vi "API Demo.vi"() -> ()   [LabVIEW 2020]
doc: "Demonstration of API useage."
uses:
  Framework/Execution API/Execution API.lvclass
panel:
  out "All Passed?":bool
  out "Output":string
  in  "Run Tests In Parallel? (T)":bool=TRUE
  in  "Tab Control":enum32{"Path", "App Instance"}(tab)
  in  "Project, Library, or Test Class Path":path
  out "error out":errorcluster
  in  "error in":errorcluster
  # "1. Select which method you want to use for finding tests to run from the API by choosing a tab in the tab control.\n2. Fill in the path to the test to run.  \n3. Run this VI."
  # "Execute all tests found in the current application instance"
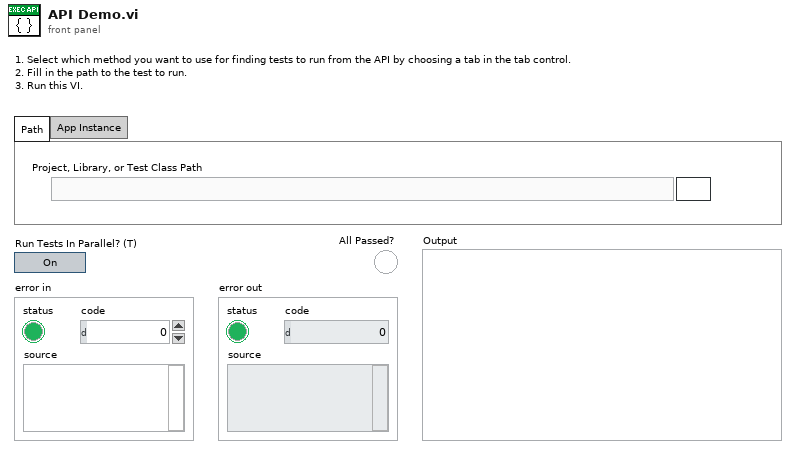
[diagram p1: front panel]
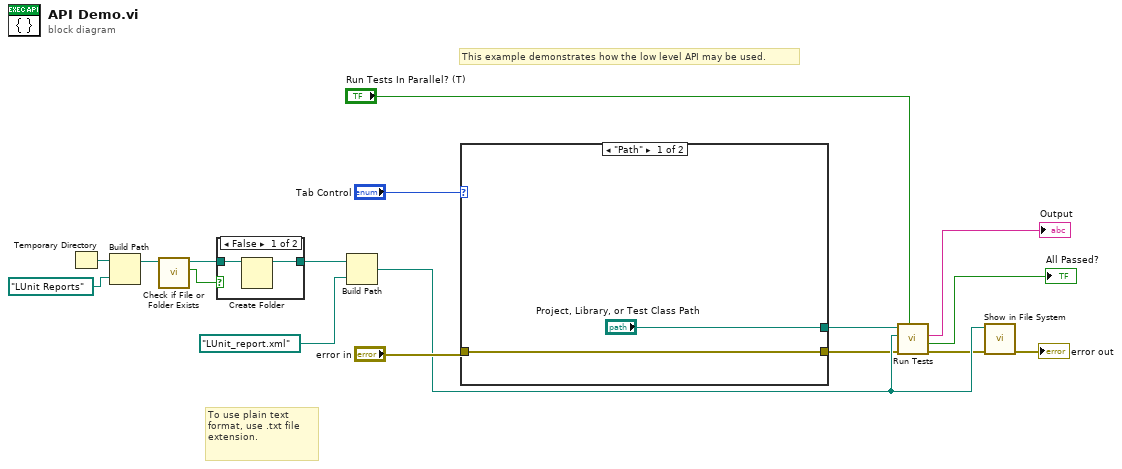
[diagram p0: block diagram]
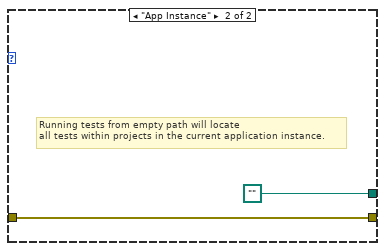
[diagram p2: hidden frame]
diagram:
  # "To use plain text format, use .txt file extension."
  # "This example demonstrates how the low level API may be used."
  n1 = Temporary Directory() -> (w12:path)
  n2 = Build Path(base path=w12, name or relative path=path "LUnit Reports") -> (appended path=w13:path)
  n3 = call <vilib>:"Check if File or Folder Exists.vi"("path"=w13) -> ("file or folder exists?"=w9:bool, "dup path"=w10:path)  [unwired: 8 in, 1 out]
  n4 = case shown="False" w9 {
    tunnel: w10 -> [w19 w20]
    tunnel: [w18 w20] -> w8
    frame False {
      n5 = Create Folder(path (use dialog)=w19) -> (created path=w18:path)  [unwired: 2 in, 2 out]
    }
    frame True {
    }
  }
  n6 = Build Path(base path=w8, name or relative path=path "LUnit_report.xml") -> (appended path=w6:path)
  n7 = case shown="\"Path\"" "Tab Control" {
    tunnel: "error in" -> [w22 w24]
    tunnel: [w22 w24] -> w3
    tunnel: ["Project, Library, or Test Class Path" path "" ("Project or Class Path")] -> w7
    frame "Path" {
    }
    frame "App Instance" {
      # "Running tests from empty path will locate\nall tests within projects in the current application instance."
    }
  }
  n8 = call "Run Tests.vi"("Run Tests In Parallel? (T)"="Run Tests In Parallel? (T)", "error in (no error)"=w3, "Report Output path"=w6, "Project, Library, or Test Class Path"=w7) -> ("error out"=w4:errorcluster, "All Passed?"=→"All Passed?":bool, "Output"=→"Output":string)  [unwired: 5 in]
  n9 = call <vilib>:"Show in File System.vi"("error in (no error)"=w4, "file or directory path"=w6) -> ("error out"=→"error out":errorcluster)  [unwired: 9 in]
